vi "calib_file.vi"() -> ()   [LabVIEW 2019]
uses:
  <vilib>/Platform/TimedLoop/XDataNode/timing_clust.ctl
  <vilib>/Platform/TimedLoop/XDataNode/nitl_modes.ctl
  <vilib>/Platform/TimedLoop/XDataNode/wakeup.ctl
  <vilib>/platform/TimedLoop/XDataNode/XDataNode.xnode
  <vilib>/Platform/TimedLoop/XDataNode/XDNodeRunTimeDep.lvlib
panel:
  in  "stop":bool
  out "[mm/pixel]":dbl
  in  "Line Length [mm]":dbl
  out "Line Length [pixel]":dbl
  out "Image Out":T1(plugin-control)
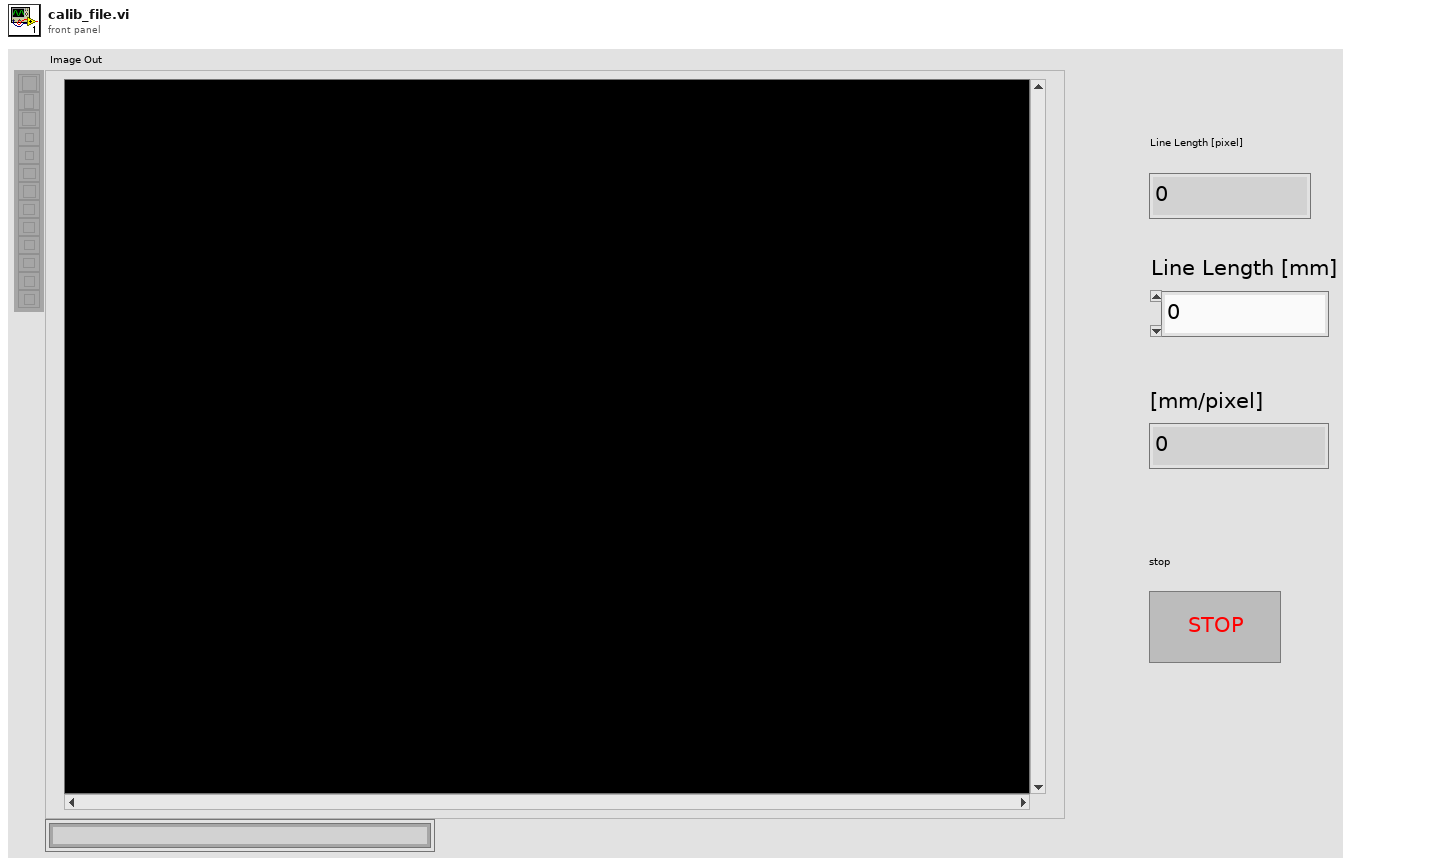
[diagram p1: front panel]
types:
  T1 = typedef "IMAQ Image.ctl" = refnum<image>
  T2 = typedef "XDNodeRunTimeDep.lvlib/timing_clust.ctl" = cluster{"Expected End [f-1]":u64, "Actual End [f-1]":u64, "Finished Late? [f-1]":bool, "Expected End [i-1]":u64, "Actual End [i-1]":u64, "Finished Late? [i-1]":bool, "Expected Start [i]":u64, "Actual Start [i]":u64, "Expected Start [f]":u64, "Actual Start [f]":u64, "Source Name":string, "Structure Name":string, "Period":i64, "Deadline":i64, "Offset":i64, "Start":i64, "Priority":i32, "Timeout":i32, "Mode":T3, "Wakeup Reason":T4, "Error":errorcluster, "Source Type":string, "Secondary Source Type":string, "Global End Time":u64, "Global Start Time":u64, "Frame Duration":u64, "Iteration Duration":u64, "Assigned CPU":i32, "I/O Scan Engine Mode":u32}
  T3 = typedef "XDNodeRunTimeDep.lvlib/nitl_modes.ctl" = enum32{"No Change", "Process missed periods, maintain original phase", "Discard missed periods, maintain original phase", "Process missed periods, ignore original phase", "Discard missed periods, ignore original phase"}
  T4 = typedef "XDNodeRunTimeDep.lvlib/wakeup.ctl" = enum32{"Normal", "Aborted", "Asynchronous wakeup", "Timing source error", "Timed loop error", "Timeout"}
  T5 = typedef "IMAQ Line" = cluster{"Start X":i32, "Start Y":i32, "End X":i32, "End Y":i32}
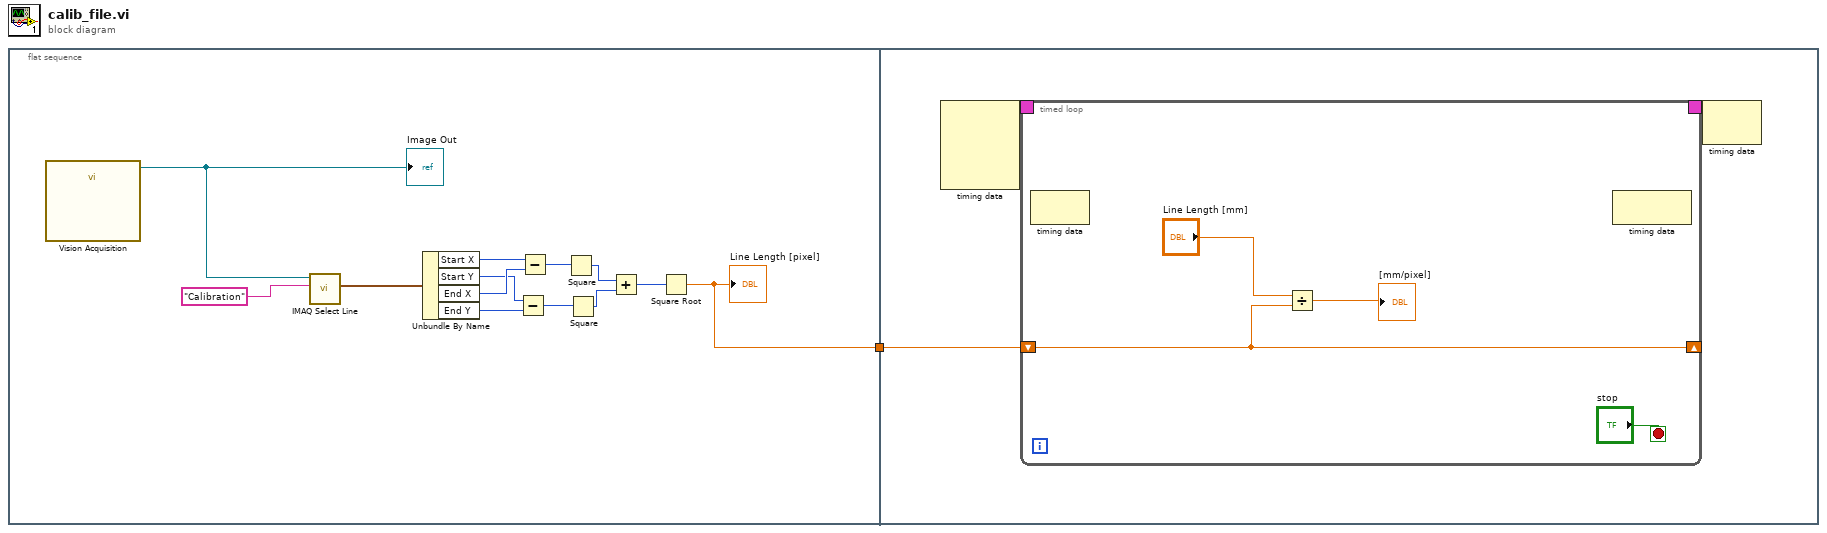
[diagram p0: block diagram]
diagram:
  n1 = flat-sequence {
    tunnel: [w14] -> w1
    tunnel: w1 -> [w17]
    frame #0 {
      n2 = call "Vision Acquisition"() -> ("Image Out"=w13:T1)  [unwired: 26 in, 1 out]
      "Image Out" <- w13
      n3 = call "IMAQ Select Line"("Prompt"="Calibration", "Image In"=w13) -> ("Line"=w12:T5)  [unwired: 6 in, 3 out]
      n4 = Unbundle By Name(w12) -> ("Start X"=w10:i32, "Start Y"=w7:i32, "End X"=w9:i32, "End Y"=w8:i32)
      n5 = Subtract(x=w7, y=w8) -> (x-y=w5:i32)
      n6 = Subtract(x=w10, y=w9) -> (x-y=w6:i32)
      n7 = Square(x=w6) -> (x^2=w4:i32)
      n8 = Square(x=w5) -> (x^2=w3:i32)
      n9 = Add(x=w4, y=w3) -> (x+y=w2:i32)
      n10 = Square Root(x=w2) -> (sqrt(x)=w14:dbl)
      "Line Length [pixel]" <- w14
    }
    frame #1 {
      n11 = node-c288() -> (w16:T2)  [unwired: 4 in]
      n12 = timed-loop {
        timing: w16 -> [_]
        timing-out: [_] -> w15
        shift-right: [w18] -> _
        shift-left: w17 -> [w18]
        stop <- "stop" stop-if-true
        n13 = node-c288() -> ()  [unwired: 1 in, 1 out]
        n14 = Divide(x="Line Length [mm]", y=w18) -> (x/y=→"[mm/pixel]":dbl)
        n15 = node-c288() -> ()  [unwired: 1 in, 1 out]
      }
      n16 = node-c288(w15) -> ()  [unwired: 1 out]
    }
  }
